vi "SBE37LivePlotting.vi"() -> ()   [LabVIEW 2020]
doc: "This example performs a serial port write and a serial port read. The parameters set for the serial port must match the parameters of the connected instrument or device. The VISA Configure Serial Port VI sets the configuration parameters. The front panel displays the controls used to configure the basic parameters, such as baud rate, data bits, and parity. The VI passes the VISA resource name to other VIs that perform operations on that VISA resource. The VISA Write function sends a command to the serial device and the VISA Read function returns data based on the command. The VISA Close function then closes the reference to the serial device. It is important to close the reference; otherwise, further communication through that port might not be possible."
uses:
  <vilib>/picture/cartesn2.llb/XY Plot Type.ctl
  d40ec6dd-3ecf-4240-bb8a-4498ac5227aa.vi
  <vilib>/Array/Sort 2D Array - Pop Stack.vi
  <vilib>/Array/Sort 2D Array - Push Stack.vi
  <vilib>/Instr/_visa.llb/VISA Configure Serial Port (Instr).vi
  <vilib>/Utility/file.llb/Read Delimited Spreadsheet (string).vi
  <vilib>/Utility/file.llb/Write Delimited Spreadsheet (string).vi
panel:
  in  "XY plot cosmetics":T2={"plot color"=16776960, "XY plot type"=enum."connected points", "baseline"=0.0} {"baseline" format="%0.2f"}
  in  "cartesian axis attributes":T3={"x minimum"=0.0, "x maximum"=0.0, "x log?"=FALSE, "x precision"=1, "x format"=enum."Decimal", "y minimum"=0.0, "y maximum"=0.0, "y log?"=FALSE, "y precision"=1, "y format"=enum."Decimal"} {"x minimum" format="%0.2f"; "x maximum" format="%0.2f"; "y minimum" format="%0.2f"; "y maximum" format="%0.2f"}
  out "Table Control":string[][](table)
  out "2D Picture":picture
  in  "error in (no error)":errorcluster
  out "?":u32
  out "Response":string
  in  "VISA resource name":refnum<visa-resource-name>="COM1"
  # "Overview: Demonstrates the use of the VISA functions to send a single command to a serial instrument and read a response.\nRequirements: NI-VISA Driver\nInstructions:\n1. Ensure the resource specified by the VISA resource name is a valid serial device.\n2. Run the VI.\n3. If your instrument recognizes the \"*IDN?\" command, it should return a Response."
  # "Note: For an example of how to perform continuous serial communication in a loop, open the Continuous Serial Write and Read.vi in the same folder as this example."
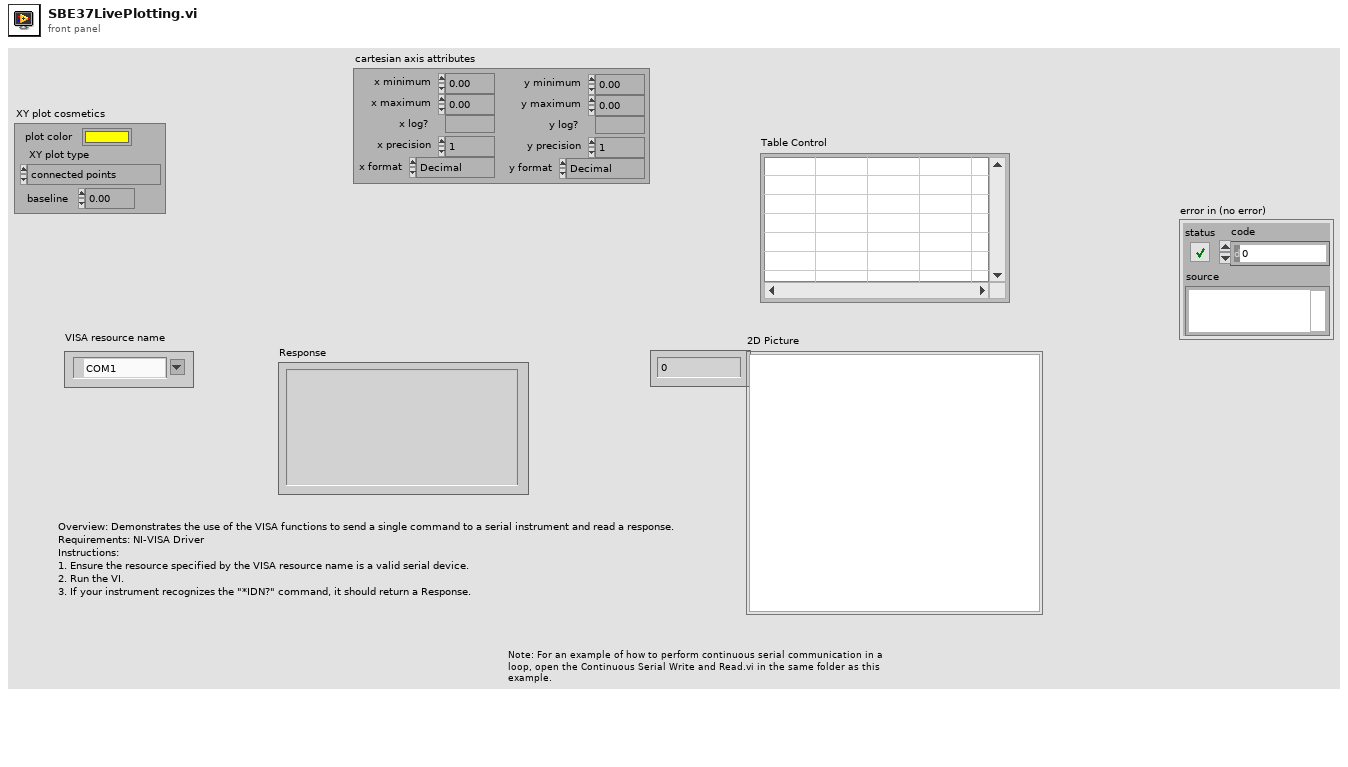
[diagram p1: front panel]
types:
  T1 = typedef "XY Plot Type.ctl" = enum16{"points", "squares", "circles", "connected points", "connected squares", "connected circles", "comb plot", "sized scatter plot", "sized-colored scatter plot", "min-max lines"}
  T2 = cluster{"plot color":u32, "XY plot type":T1, "baseline":dbl}
  T3 = cluster{"x minimum":dbl, "x maximum":dbl, "x log?":bool, "x precision":u8, "x format":enum8{"Decimal", "Scientific", "Engineering", "Binary", "Octal", "Hex"}, "y minimum":dbl, "y maximum":dbl, "y log?":bool, "y precision":u8, "y format":enum8{"Decimal", "Scientific", "Engineering", "Binary", "Octal", "Hex"}}
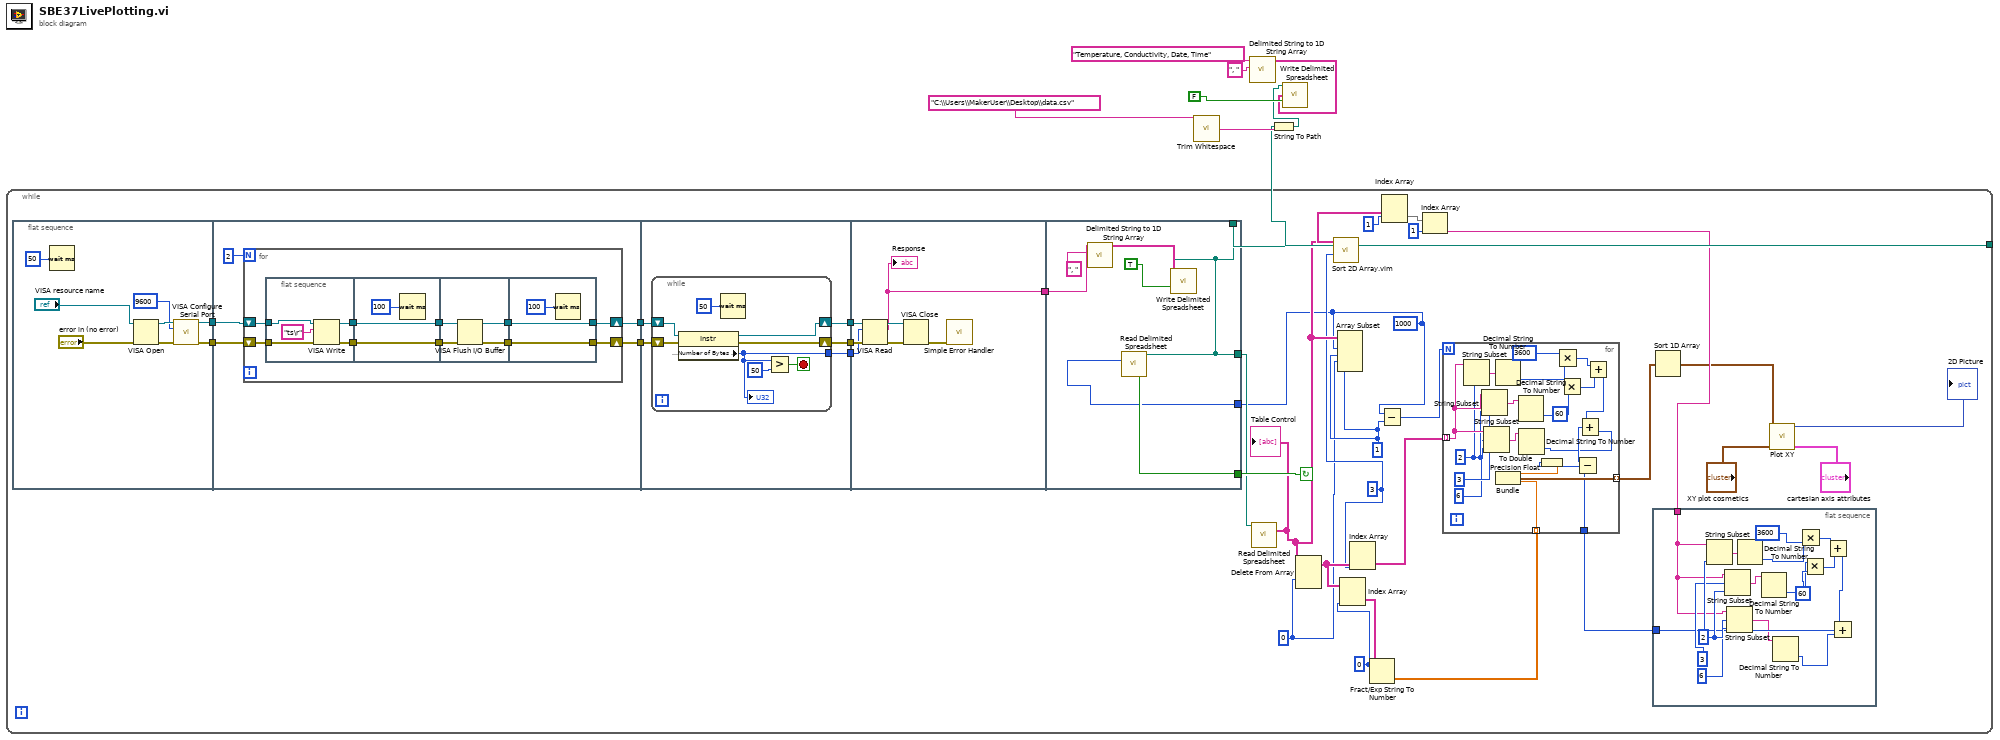
[diagram p0: block diagram]
diagram:
  n1 = call <vilib>:"Trim Whitespace.vi"("string"="C:\\Users\\MakerUser\\Desktop\\data.csv") -> ("trimmed string"=w6:string)  [unwired: 1 in]
  n2 = call <vilib>:"Delimited String to 1D String Array.vi"("delimiter"=", ", "delimited string"="Temperature, Conductivity, Date, Time") -> ("string array"=w3:string[])  [unwired: 9 in]
  n3 = String To Path(string=w6) -> (path=w1:path)
  n4 = while {
    tunnel: w1 -> [w32]
    stop <- w31 continue-if-true
    w8 = 1000
    w11 = 1
    w14 = 3
    w15 = 0
    w10 = 0
    n5 = flat-sequence {
      tunnel: [w79] -> w40
      tunnel: [w78] -> w39
      tunnel: w40 -> [w90]
      tunnel: w39 -> [w89]
      tunnel: [w87] -> w38
      tunnel: [w86] -> w37
      tunnel: w38 -> [w120]
      tunnel: w37 -> [w119]
      tunnel: [w118] -> w36
      tunnel: [w117] -> w35
      tunnel: [w116] -> w34
      tunnel: w36 -> [w135]
      tunnel: w35 -> [w134]
      tunnel: w34 -> [w133]
      tunnel: [w129] -> w33
      tunnel: w33 -> [w142]
      tunnel: w32 -> [w137]
      tunnel: [w138] -> w31
      tunnel: [w137] -> w9
      tunnel: w8 -> [w136]
      frame #0 {
        n6 = Wait (ms)(milliseconds to wait=50) -> ()  [unwired: 1 out]
        n7 = VISA Open(error in (no error)="error in (no error)", VISA resource name="VISA resource name") -> (VISA resource name=w83:refnum<visa-resource-name>, error out=w82:errorcluster)  [unwired: 3 in]
        n8 = call-poly "VISA Configure Serial Port"("VISA resource name"=w83, "baud rate (9600)"=u32 9600, "error in (no error)"=w82) -> ("VISA resource name out"=w79:refnum<visa-resource-name>, "error out"=w78:errorcluster)  [unwired: 6 in, 5 out]
      }
      frame #1 {
        n9 = for {
          N: 2 -> [_]
          shift-right: [w93] -> w87
          shift-left: w90 -> [w92]
          shift-right: [w94] -> w86
          shift-left: w89 -> [w91]
          n10 = flat-sequence {
            tunnel: w92 -> [w104]
            tunnel: w91 -> [w103]
            tunnel: [w102] -> w100
            tunnel: [w101] -> w97
            tunnel: w100 -> [w108]
            tunnel: [w108] -> w99
            tunnel: [w107] -> w98
            tunnel: w97 -> [w107]
            tunnel: w99 -> [w112]
            tunnel: w98 -> [w111]
            tunnel: [w110] -> w96
            tunnel: [w109] -> w95
            tunnel: [w115] -> w93
            tunnel: w96 -> [w115]
            tunnel: [w114] -> w94
            tunnel: w95 -> [w114]
            frame #0 {
              n11 = VISA Write(VISA resource name=w104, write buffer="ts\r", error in (no error)=w103) -> (VISA resource name out=w101:refnum<visa-resource-name>, error out=w102:errorcluster)  [unwired: 1 out]
            }
            frame #1 {
              n12 = Wait (ms)(milliseconds to wait=u32 100) -> ()  [unwired: 1 out]
            }
            frame #2 {
              n13 = VISA Flush I/O Buffer(VISA resource name=w111, error in (no error)=w112) -> (VISA resource name out=w110:refnum<visa-resource-name>, error out=w109:errorcluster)  [unwired: 1 in]
            }
            frame #3 {
              n14 = Wait (ms)(milliseconds to wait=u32 100) -> ()  [unwired: 1 out]
            }
          }
        }
      }
      frame #2 {
        n15 = while {
          tunnel: [w123] -> w116
          shift-right: [w126] -> w117
          shift-left: w119 -> [w121]
          shift-right: [w127] -> w118
          shift-left: w120 -> [w122]
          stop <- w124 stop-if-true
          n16 = property class="Instr"(reference=w122, error in=w121) -> (reference out=w127:refnum<visa-resource-name>, error out=w126:errorcluster, "Serial Settings:Number of Bytes at Serial Port"=w123:u32)
          "?" <- w123
          n17 = Wait (ms)(milliseconds to wait=50) -> ()  [unwired: 1 out]
          n18 = Greater?(x=w123, y=u32 50 ("Serial Settings:Number of Bytes at Serial Port")) -> (0:w124:bool)
        }
      }
      frame #3 {
        n19 = VISA Read(VISA resource name=w135, byte count=w133, error in (no error)=w134) -> (VISA resource name out=w131:refnum<visa-resource-name>, read buffer=w129:string, error out=w130:errorcluster)  [unwired: 1 out]
        "Response" <- w129
        n20 = VISA Close(VISA resource name=w131, error in (no error)=w130) -> (error out=w132:errorcluster)
        n21 = call <vilib>:"Simple Error Handler.vi"("error in (no error)"=w132) -> ()  [unwired: 1 in, 8 out]
      }
      frame #4 {
        n22 = call <vilib>:"Delimited String to 1D String Array.vi"("delimiter"=", ", "delimited string"=w142) -> ("string array"=w139:string[])  [unwired: 9 in]
        n23 = call-poly <vilib>:"Read Delimited Spreadsheet.vi"("file path (dialog if empty)"=w137, "number of rows (all:-1)"=w136) -> ("EOF?"=w138:bool)  [unwired: 8 in, 5 out]
        n24 = call-poly <vilib>:"Write Delimited Spreadsheet.vi"("file path (dialog if empty)"=w137, "1D data"=w139, "append to file? (new file:F)"=TRUE) -> ()  [unwired: 11 in, 2 out]
      }
    }
    n25 = call-poly <vilib>:"Read Delimited Spreadsheet.vi"("file path (dialog if empty)"=w9) -> ("all rows"=w25:string[][])  [unwired: 9 in, 5 out]
    "Table Control" <- w25
    n26 = Delete From Array(array=w25, index (row)=w10) -> (array with subset deleted=w16:string[][])  [unwired: 2 in, 1 out]
    n27 = call "Sort 2D Array.vim"("index"=w14, "2D array"=w25) -> ("sorted 2D array"=w26:string[][])  [unwired: 8 in, 1 out]
    n28 = Array Subset(array=w25, index (row)=w8, length (row)=w11, index (col)=w10, length (col)=w11) -> ()  [unwired: 1 out]
    n29 = Index Array(array=w16, index (col)=w15) -> (element=w27:string[])  [unwired: 1 in]
    n30 = Index Array(array=w16, index (col)=w14) -> (element=w18:string[])  [unwired: 1 in]
    n31 = Fract/Exp String To Number(string=w27, offset=w15) -> (number=w28:dbl[])  [unwired: 2 in, 1 out]
    n32 = Subtract(x=w8, y=w11) -> (x-y=w17:i32)
    n33 = Index Array(array=w26, index (row)=1) -> (element=w23:string[])  [unwired: 1 in]
    n34 = Index Array(array=w23, index=1) -> (element=w24:string)
    n35 = for {
      N: w17 -> [_]
      tunnel: w18 -> [w75] mode=indexing
      tunnel: [w77] -> w20 mode=indexing
      tunnel: w22 -> [w64]
      tunnel: w28 -> [w57] mode=indexing
      w74 = 2
      n36 = String Subset(string=w75, length (rest)=w74) -> (substring=w63:string)  [unwired: 1 in]
      n37 = String Subset(string=w75, offset (0)=3, length (rest)=w74) -> (substring=w62:string)
      n38 = String Subset(string=w75, offset (0)=6, length (rest)=w74) -> (substring=w61:string)
      n39 = Decimal String To Number(string=w63) -> (number=w59:i32)  [unwired: 2 in, 1 out]
      n40 = Decimal String To Number(string=w62) -> (number=w58:i32)  [unwired: 2 in, 1 out]
      n41 = Decimal String To Number(string=w61) -> (number=w60:i32)  [unwired: 2 in, 1 out]
      n42 = Multiply(x=w59, y=3600) -> (x*y=w69:i32)
      n43 = Multiply(x=w58, y=60) -> (x*y=w68:i32)
      n44 = Add(x=w69, y=w68) -> (x+y=w67:i32)
      n45 = Add(x=w67, y=w60) -> (x+y=w66:i32)
      n46 = Subtract(x=w66, y=w64) -> (x-y=w65:i32)
      n47 = To Double Precision Float(number=w65) -> (double precision float=w76:dbl)
      n48 = Bundle(w76, "String"=w57) -> (w77:cluster{dbl, "String":dbl})  [unwired: 1 in]
    }
    n49 = flat-sequence {
      tunnel: [w48] -> w22
      tunnel: w24 -> [w47]
      frame #0 {
        w51 = 2
        n50 = String Subset(string=w47, length (rest)=w51) -> (substring=w46:string)  [unwired: 1 in]
        n51 = String Subset(string=w47, offset (0)=3, length (rest)=w51) -> (substring=w41:string)
        n52 = String Subset(string=w47, offset (0)=6, length (rest)=w51) -> (substring=w44:string)
        n53 = Decimal String To Number(string=w46) -> (number=w45:i32)  [unwired: 2 in, 1 out]
        n54 = Decimal String To Number(string=w41) -> (number=w42:i32)  [unwired: 2 in, 1 out]
        n55 = Decimal String To Number(string=w44) -> (number=w43:i32)  [unwired: 2 in, 1 out]
        n56 = Multiply(x=w45, y=3600) -> (x*y=w56:i32)
        n57 = Multiply(x=w42, y=60) -> (x*y=w55:i32)
        n58 = Add(x=w56, y=w55) -> (x+y=w54:i32)
        n59 = Add(x=w54, y=w43) -> (x+y=w48:i32)
      }
    }
    n60 = Sort 1D Array(array=w20) -> (sorted array=w21:cluster{dbl, "String":dbl}[])
    n61 = call <vilib>:"Plot XY.vi"("data"=w21, "cartesian axis attributes"="cartesian axis attributes", "XY plot cosmetics"="XY plot cosmetics") -> ("new picture"=→"2D Picture":picture)  [unwired: 12 in]
  }
  n62 = call-poly <vilib>:"Write Delimited Spreadsheet.vi"("file path (dialog if empty)"=w1, "1D data"=w3, "append to file? (new file:F)"=FALSE) -> ()  [unwired: 11 in, 2 out]
